vi "analog_trigger_raw.vi"(0 "Triggered?":bool, 1 "Condition":T1(ring), 2 "Level":sgl, 3 "Window Amplitude":sgl step=0.1 format="%0.2f", 7 "Initialized Data Array":i16[](array[numeric]) caption="Old Data Array", 9 "Input Raw Data":i16[](array[numeric]), 11 "Pretrigger Samples":i32, 12 "Index of Condition Channel":i32, 14 "Force Restart":bool) -> (4 "Trigger Out":bool, 6 "Output Data (Scaled)":i16[](array[numeric]), 8 "Raw Data Out":i16[](array[numeric]), 10 "# Pretrigger Samples":i32, 15 "Pre-Trigger Error":bool caption="Error \n(Triggered before\n pretrigger samples\n were acquired)")   [LabVIEW 2013]
doc: "1. Description\n\nThis VI was originally intended to be part of the Acq&Graph Voltage - Analog Software Trigger (Scaled).vi NI-DAQmx example, acting as a SubVI to detect the Analog Software Trigger."
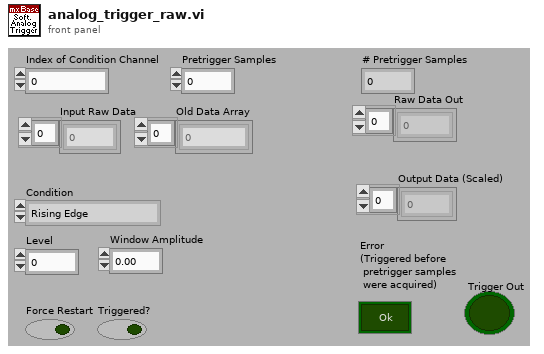
[diagram p1: front panel]
types:
  T1 = enum16{"Rising Edge", "Falling Edge", "Above Level", "Below Level", "When Inside Window", "When Outside Window"}
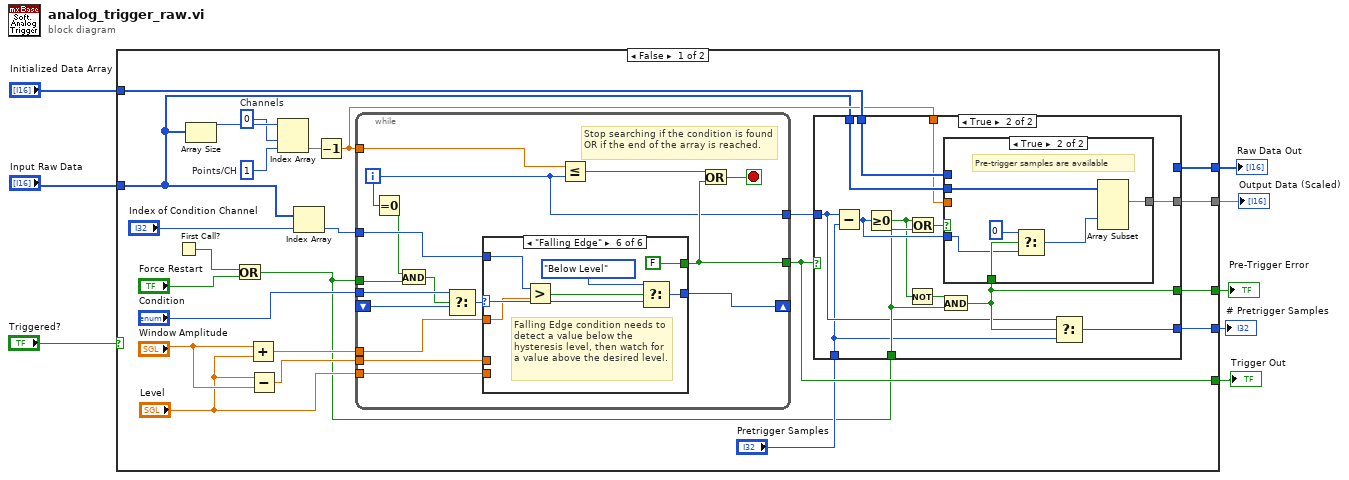
[diagram p0: block diagram]
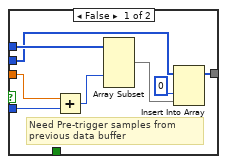
[diagram p3: hidden frame]
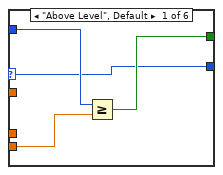
[diagram p4: hidden frame]
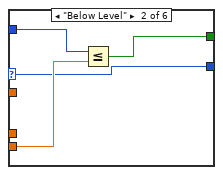
[diagram p5: hidden frame]
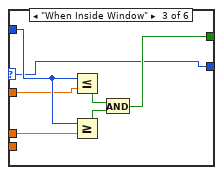
[diagram p6: hidden frame]
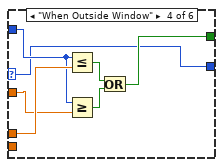
[diagram p7: hidden frame]
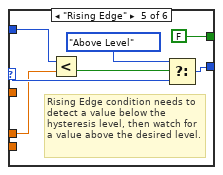
[diagram p8: hidden frame]
diagram:
  n1 = case shown="False" "Triggered?" {
    selector: "Triggered?" -> [_ w114]
    tunnel: "Input Raw Data" -> [w11 w113]
    tunnel: "Initialized Data Array" -> [w21 _]
    tunnel: [w25 w113] -> w5
    tunnel: [w24 w114] -> w4
    tunnel: [w18 _] -> w3
    tunnel: [w17 _] -> w2
    tunnel: [w15 _] -> w1
    frame False {
      w27 = 0  # Channels
      w28 = 1  # Points/CH
      n2 = First Call?() -> (First Call?: T/F=w16:bool)
      n3 = Array Size(array=w11) -> (size(s)=w29:i32)
      n4 = Or(x=w16, y="Force Restart") -> (x .or. y?=w9:bool)
      n5 = Add(x="Window Amplitude", y="Level") -> (x+y=w12:sgl)
      n6 = Subtract(x="Level", y="Window Amplitude") -> (x-y=w14:sgl)
      n7 = Index Array(array=w29, index #1=w27, index #2=w28) -> (element #2=w20)  [unwired: 1 out]
      n8 = Index Array(array=w11, index="Index of Condition Channel") -> (element=w32:i16)
      n9 = Decrement(x=w20) -> (x-1=w19:dbl)
      n10 = while {
        tunnel: w32 -> [w75]
        tunnel: "Level" -> [w76]
        tunnel: w14 -> [w74]
        tunnel: w12 -> [w73]
        tunnel: w19 -> [w61]
        tunnel: [w66] -> w24
        tunnel: [w65] -> w26
        shift-right: [w70] -> _
        shift-left: _ -> [w68]
        tunnel: "Condition" -> [w69]
        tunnel: w9 -> [w62]
        i -> [w65]
        stop <- w71 stop-if-true
        # "Stop searching if the condition is found OR if the end of the array is reached."
        n11 = Equal To 0?(x=w65) -> (x = 0?=w64:bool)
        n12 = And(x=w64, y=w62) -> (x .and. y?=w63:bool)
        n13 = Select(t=w69, s=w63, f=w68) -> (s? t:f=w67:T1)
        n14 = case shown="\"Falling Edge\"" w67 {
          selector: w67 -> [w77 w81 w85 w92 w102 w109]
          tunnel: w75 -> [w80 w84 w91 w97 w103 w110]
          tunnel: w76 -> [w79 w83 _ _ _ _]
          tunnel: [w78 w82 w86 w93 FALSE FALSE] -> w66
          tunnel: w74 -> [_ _ w90 w98 w99 _]
          tunnel: w73 -> [_ _ w89 w96 _ w106]
          tunnel: [w77 w81 w85 w92 w100 w107] -> w70
          frame "Above Level", Default {
            n15 = Greater Or Equal?(x=w80, y=w79) -> (x >= y?=w78:bool)
          }
          frame "Below Level" {
            n16 = Less Or Equal?(x=w84, y=w83) -> (x <= y?=w82:bool)
          }
          frame "When Inside Window" {
            n17 = Less Or Equal?(x=w91, y=w89) -> (x <= y?=w87:bool)
            n18 = Greater Or Equal?(x=w91, y=w90) -> (x >= y?=w88:bool)
            n19 = And(x=w87, y=w88) -> (x .and. y?=w86:bool)
          }
          frame "When Outside Window" {
            n20 = Less Or Equal?(x=w97, y=w98) -> (x <= y?=w95:bool)
            n21 = Greater Or Equal?(x=w97, y=w96) -> (x >= y?=w94:bool)
            n22 = Or(x=w95, y=w94) -> (x .or. y?=w93:bool)
          }
          frame "Rising Edge" {
            # "Rising Edge condition needs to detect a value below the hysteresis level, then watch for a value above the desired level."
            n23 = Less?(x=w103, y=w99) -> (x < y?=w101:bool)
            n24 = Select(t=T1."Above Level" ("Condition"), s=w101, f=w102) -> (s? t:f=w100:T1)
          }
          frame "Falling Edge" {
            # "Falling Edge condition needs to detect a value below the hysteresis level, then watch for a value above the desired level."
            n25 = Greater?(x=w110, y=w106) -> (0:w108:bool)
            n26 = Select(t=T1."Below Level" ("Condition"), s=w108, f=w109) -> (s? t:f=w107:T1)
          }
        }
        n27 = Less Or Equal?(x=w61, y=w65) -> (x <= y?=w72:bool)
        n28 = Or(x=w72, y=w66) -> (x .or. y?=w71:bool)
      }
      n29 = case shown="True" w24 {
        tunnel: w11 -> [w33 w45]
        tunnel: w26 -> [_ w37]
        tunnel: [_ w34] -> w25
        tunnel: "Pretrigger Samples" -> [_ w36]
        tunnel: w21 -> [_ w44]
        tunnel: w19 -> [_ w43]
        tunnel: [w33 _] -> w18
        tunnel: w9 -> [_ w41]
        tunnel: [_ w38] -> w17
        tunnel: [_ w35] -> w15
        frame False {
          # "The trigger condition was not found in the current data buffer."
        }
        frame True {
          n30 = Subtract(x=w37, y=w36) -> (x-y=w46:i32)
          n31 = Greater Or Equal To 0?(x=w46) -> (x >= 0?=w39:bool)
          n32 = Not(x=w39) -> (.not. x?=w40:bool)
          n33 = Or(x=w39, y=w41) -> (x .or. y?=w42:bool)
          n34 = And(x=w40, y=w41) -> (x .and. y?=w38:bool)
          n35 = case shown="True" w42 {
            tunnel: [w53 w60] -> w34
            tunnel: w46 -> [w47 w57]
            tunnel: w45 -> [w51 w59]
            tunnel: w44 -> [w54 _]
            tunnel: w43 -> [w48 _]
            tunnel: w38 -> [_ w58]
            frame False {
              # "Need Pre-trigger samples from previous data buffer"
              n36 = Add(x=w48, y=w47) -> (x+y=w52:i32)
              n37 = Array Subset(array=w54, index (col)=w52) -> (w50:i16[])  [unwired: 3 in]
              n38 = Insert Into Array(array=w51, index (col)=0 ("index (row)"), new element=w50) -> (w53:i16[])  [unwired: 1 in]
            }
            frame True {
              # "Pre-trigger samples are available"
              n39 = Select(t=0, s=w58, f=w57) -> (s? t:f=w56:i32)
              n40 = Array Subset(array=w59, index (col)=w56) -> (w60:i16[])  [unwired: 3 in]
            }
          }
          n41 = Select(t=w37, s=w38, f=w36) -> (s? t:f=w35:i32)
        }
      }
    }
    frame True {
      # "A trigger has already occurred, no need to monitor the data."
    }
  }
  "Output Data (Scaled)" <- w5
  "Trigger Out" <- w4
  "Raw Data Out" <- w3
  "Pre-Trigger Error" <- w2
  "# Pretrigger Samples" <- w1
